vi "Get Server Version.vi"(11 "Machine Name":string="hybridcryomac.ad.magnet.fsu.edu") -> (1 "LV Version":string, 2 "Target LV Version #":T1, 3 "Open LabVIEW Ports":u16[](array[numeric]))   [LabVIEW 2019]
uses:
  Sub Controls/LV Versions Enum.ctl
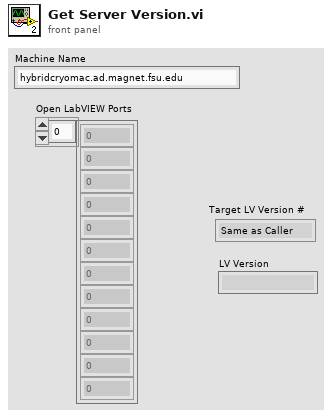
[diagram p1: front panel]
types:
  T1 = typedef "LV Versions Enum.ctl" = enum16{"Same as Caller", "8.0", "8.20", "8.5", "8.6", "9.0", "10.0", "11.0", "12.0", "13.0", "14.0", "15.0", "16.0", "17.0", "18.0", "19.0", "20.0"}
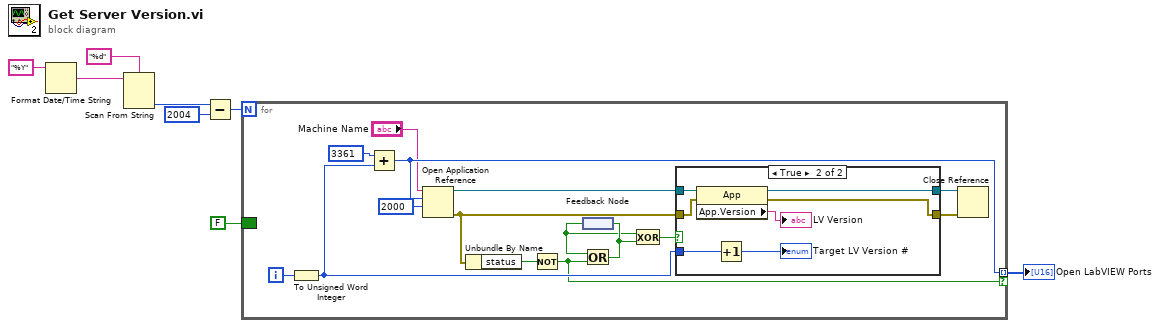
[diagram p0: block diagram]
diagram:
  n1 = Format Date/Time String(time format string (%c)="%Y") -> (date/time string=w7:string)  [unwired: 2 in]
  n2 = Scan From String(format string="%d", input string=w7) -> (output 1=w5:i32)  [unwired: 3 in, 3 out]
  n3 = Subtract(x=w5, y=2004) -> (x-y=w3:i32)
  n4 = for {
    N: w3 -> [_]
    tunnel: [w20] -> w2 mode=indexing if=w13
    border: FALSE -> [_]
    i -> [w23]
    n5 = To Unsigned Word Integer(number=w23) -> (unsigned 16bit integer=w14:u16)
    n6 = Add(x=u16 3361, y=w14) -> (x+y=w20:u16)
    n7 = Open Application Reference(9:2000 ("timeout ms (60000)"), 10:w20, 11:"Machine Name") -> (0:w16:errorcluster, 3:w18:refnum<vi>)  [unwired: 1 in]
    n8 = Unbundle By Name(w16) -> ("status"=w21:bool)
    n9 = Not(x=w21) -> (.not. x?=w13:bool)
    n10 = feedback #1() -> (w10:bool)
    n11 = Or(x=w10, y=w13) -> (x .or. y?=w11:bool)
    n12 = feedback-in #1(w11) -> ()
    n13 = Exclusive Or(1:w11, 2:w10) -> (0:w12:bool)
    n14 = case shown="True" w12 {
      tunnel: w18 -> [w25 w31]
      tunnel: [w25 w30] -> w17
      tunnel: w16 -> [w24 w29]
      tunnel: [w24 w28] -> w15
      tunnel: w14 -> [_ w27]
      frame False {
      }
      frame True {
        n15 = property class="App"(reference=w31, error in=w29) -> (reference out=w30:refnum<vi>, error out=w28:errorcluster, "App.Version"=→"LV Version":string)
        n16 = Increment(x=w27) -> (x+1=→"Target LV Version #":u16)
      }
    }
    n17 = Close Reference(reference=w17, error in (no error)=w15) -> ()  [unwired: 1 out]
  }
  "Open LabVIEW Ports" <- w2
